vi "GetDACRS232 V1_2.vi"(3 "error in (no error)":errorcluster, 4 "VISA resource name IN":refnum<visa-resource-name>="COM1") -> (0 "error out":errorcluster, 1 "VISA resource name OUT":refnum<visa-resource-name>="COM1", 2 "DAC data out\n(hexadecimaal)":u16[](array[numeric]) format="%x")   [LabVIEW 2011]
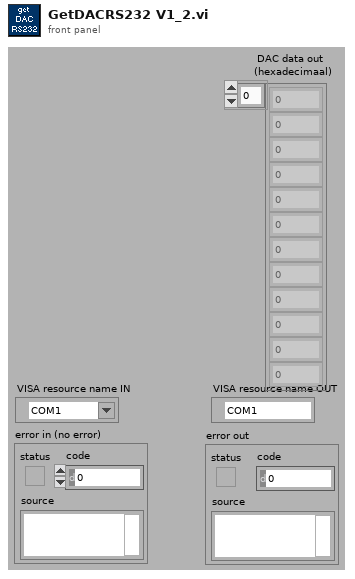
[diagram p1: front panel]
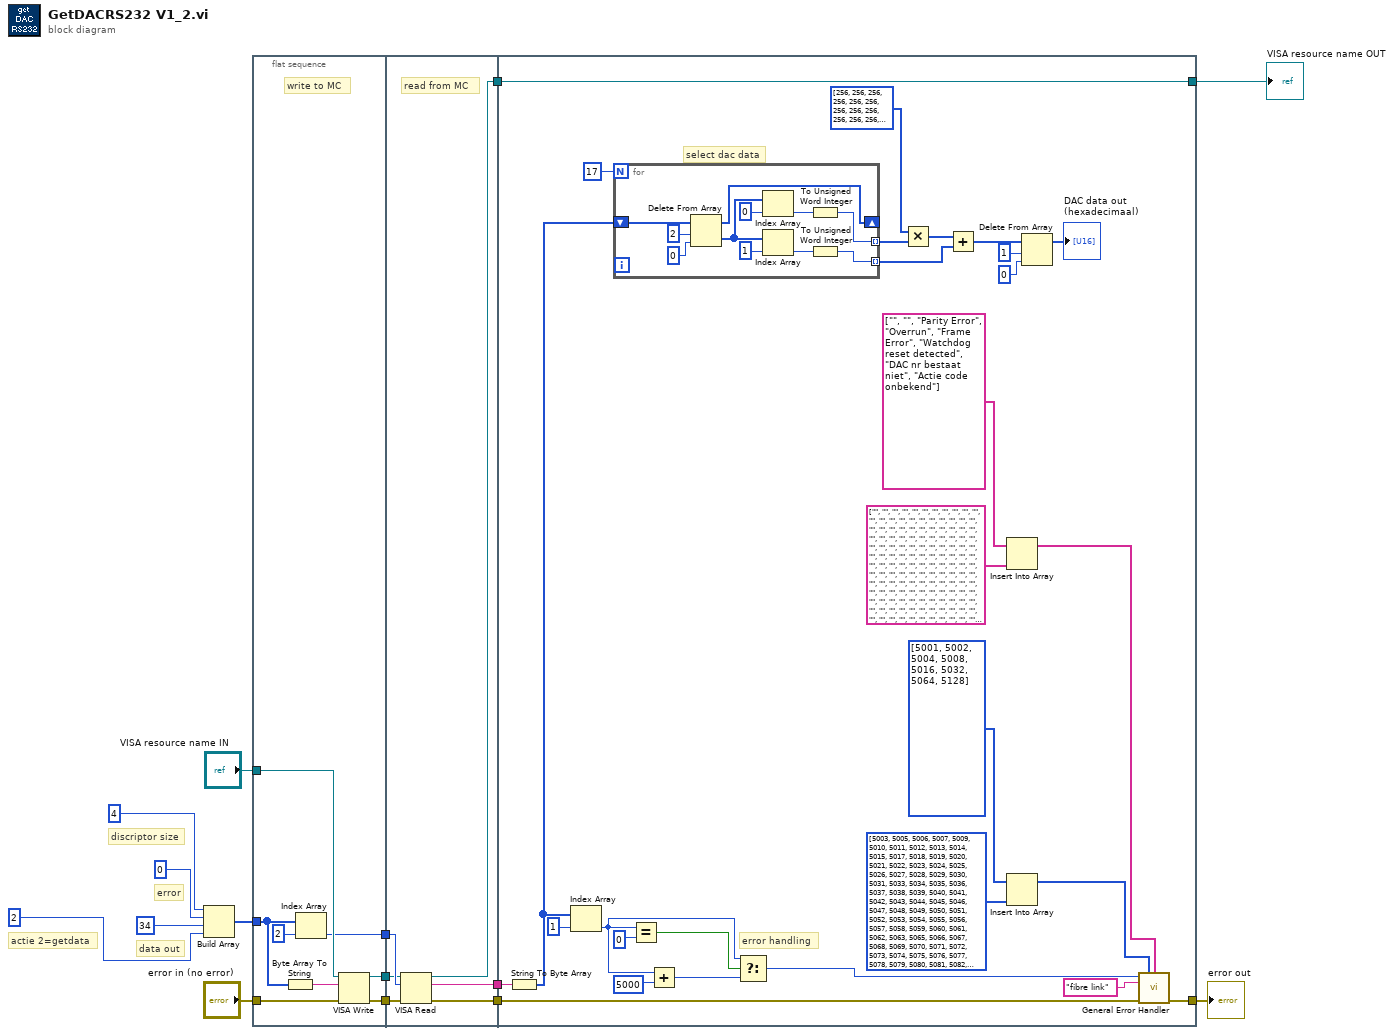
[diagram p0: block diagram]
diagram:
  # "discriptor size"
  # "error"
  # "data out"
  # "actie 2=getdata"
  n1 = Build Array(u8 4 ("array"), u8 0 ("element"), u8 34 ("element"), u8 2 ("element")) -> (w8:u8[])
  n2 = flat-sequence {
    tunnel: "VISA resource name IN" -> [w22]
    tunnel: [w20] -> w15
    tunnel: [w17] -> w14
    tunnel: [w18] -> w13
    tunnel: w8 -> [w19]
    tunnel: "error in (no error)" -> [w16]
    tunnel: w15 -> [w29]
    tunnel: w14 -> [w28]
    tunnel: w13 -> [w27]
    tunnel: [w26] -> w5
    tunnel: [w25] -> w4
    tunnel: [w24] -> w3
    tunnel: [w38] -> w1
    tunnel: w5 -> [w41]
    tunnel: w4 -> [w40]
    tunnel: [w39] -> w2
    tunnel: w3 -> [w39]
    frame #0 {
      # "write to MC"
      n3 = Byte Array To String(unsigned byte array=w19) -> (string=w23:string)
      n4 = Index Array(array=w19, index=2) -> (element=w20:u8)
      n5 = VISA Write(VISA resource name=w22, write buffer=w23, error in (no error)=w16) -> (VISA resource name out=w17:refnum<visa-resource-name>, error out=w18:errorcluster)  [unwired: 1 out]
    }
    frame #1 {
      # "read from MC"
      n6 = VISA Read(VISA resource name=w28, byte count=w29, error in (no error)=w27) -> (VISA resource name out=w24:refnum<visa-resource-name>, read buffer=w25:string, error out=w26:errorcluster)  [unwired: 1 out]
    }
    frame #2 {
      # "select dac data"
      # "error handling"
      n7 = String To Byte Array(string=w40) -> (unsigned byte array=w37:u8[])
      n8 = Index Array(array=w37, index=1) -> (element=w56:u8)
      n9 = for {
        N: 17 -> [_]
        shift-right: [w62] -> _
        shift-left: w37 -> [w66]
        tunnel: [w61] -> w45 mode=indexing
        tunnel: [w58] -> w42 mode=indexing
        n10 = Delete From Array(array=w66, length=2, index=0) -> (deleted portion=w64:u8[], array with subset deleted=w62:u8[])
        n11 = Index Array(array=w64, index=0) -> (element=w59:u8)
        n12 = Index Array(array=w64, index=1) -> (element=w60:u8)
        n13 = To Unsigned Word Integer(number=w59) -> (unsigned 16bit integer=w58:u16)
        n14 = To Unsigned Word Integer(number=w60) -> (unsigned 16bit integer=w61:u16)
      }
      n15 = Equal?(x=w56, y=u8 0) -> (x = y?=w55:bool)
      n16 = Add(x=w56, y=u32 5000) -> (x+y=w53:u32)
      n17 = Select(t=w56, s=w55, f=w53) -> (s? t:f=w54:u32)
      n18 = Multiply(x=u16[] [256, 256, 256, 256, 256, 256, 256, 256, 256, 256, 256, 256, 256, 256, 256, 256, 256], y=w42) -> (x*y=w44:u16[])
      n19 = Add(x=w44, y=w45) -> (x+y=w46:u16[])
      n20 = Insert Into Array(array=string[] ["", "", "Parity Error", "Overrun", "Frame Error", "Watchdog reset detected", "DAC nr bestaat niet", "Actie code onbekend"] ("[user-defined descriptions]"), new element=string[] ["", "", "", "", "", "", "", "", "", "", "", "", "", "", "", "", "", "", "", "", "", "", "", "", "", "", "", "", "", "", "", "", "", "", "", "", "", "", "", "", "", "", "", "", "", "", "", "", "", "", "", "", "", "", "", "", "", "", "", "", "", "", "", "", "", "", "", "", "", "", "", "", "", "", "", "", "", "", "", "", "", "", "", "", "", "", "", "", "", "", "", "", "", "", "", "", "", "", "", "", "", "", "", "", "", "", "", "", "", "", "", "", "", "", "", "", "", "", "", "", "", "", "", "", "", "", "", "", "", "", "", "", "", "", "", "", "", "", "", "", "", "", "", "", "", "", "", "", "", "", "", "", "", "", "", "", "", "", "", "", "", "", "", "", "", "", "", "", "", "", "", "", "", "", "", "", "", "", "", "", "", "", "", "", "", "", "", "", "", "", "", "", "", "", "", "", "", "", "", "", "", "", "", "", "", "", "", "", "", "", "", "", "", "", "", "", "", "", "", "", "", "", "", "", "", "", "", "", "", "", "", "", "", "", "", "", "", "", "", "", "", "", "", "", "", "", "", "", "", "", "", "", "", "", "", "", "", "", "", "", "", "", "", "", "", "", "", "", "", "", "", "", "", "", "", "", "", "", "", "", "", "", "", "", "", "", "", "", "", "", "", "", "", "", "", "", "", "", ""] ("Array 2")) -> (w30:string[])  [unwired: 1 in]
      n21 = Insert Into Array(array=i32[] [5001, 5002, 5004, 5008, 5016, 5032, 5064, 5128] ("[user-defined codes]"), new element=i32[] [5003, 5005, 5006, 5007, 5009, 5010, 5011, 5012, 5013, 5014, 5015, 5017, 5018, 5019, 5020, 5021, 5022, 5023, 5024, 5025, 5026, 5027, 5028, 5029, 5030, 5031, 5033, 5034, 5035, 5036, 5037, 5038, 5039, 5040, 5041, 5042, 5043, 5044, 5045, 5046, 5047, 5048, 5049, 5050, 5051, 5052, 5053, 5054, 5055, 5056, 5057, 5058, 5059, 5060, 5061, 5062, 5063, 5065, 5066, 5067, 5068, 5069, 5070, 5071, 5072, 5073, 5074, 5075, 5076, 5077, 5078, 5079, 5080, 5081, 5082, 5083, 5084, 5085, 5086, 5087, 5088, 5089, 5090, 5091, 5092, 5093, 5094, 5095, 5096, 5097, 5098, 5099, 5100, 5101, 5102, 5103, 5104, 5105, 5106, 5107, 5108, 5109, 5110, 5111, 5112, 5113, 5114, 5115, 5116, 5117, 5118, 5119, 5120, 5121, 5122, 5123, 5124, 5125, 5126, 5127, 5129, 5130, 5131, 5132, 5133, 5134, 5135, 5136, 5137, 5138, 5139, 5140, 5141, 5142, 5143, 5144, 5145, 5146, 5147, 5148, 5149, 5150, 5151, 5152, 5153, 5154, 5155, 5156, 5157, 5158, 5159, 5160, 5161, 5162, 5163, 5164, 5165, 5166, 5167, 5168, 5169, 5170, 5171, 5172, 5173, 5174, 5175, 5176, 5177, 5178, 5179, 5180, 5181, 5182, 5183, 5184, 5185, 5186, 5187, 5188, 5189, 5190, 5191, 5192, 5193, 5194, 5195, 5196, 5197, 5198, 5199, 5200, 5201, 5202, 5203, 5204, 5205, 5206, 5207, 5208, 5209, 5210, 5211, 5212, 5213, 5214, 5215, 5216, 5217, 5218, 5219, 5220, 5221, 5222, 5223, 5224, 5225, 5226, 5227, 5228, 5229, 5230, 5231, 5232, 5233, 5234, 5235, 5236, 5237, 5238, 5239, 5240, 5241, 5242, 5243, 5244, 5245, 5246, 5247, 5248, 5249, 5250, 5251, 5252, 5253, 5254, 5255, 5256, 5257, 5258, 5259, 5260, 5261, 5262, 5263, 5264, 5265, 5266, 5267, 5268, 5269, 5270, 5271, 5272, 5273, 5274, 5275, 5276, 5277, 5278, 5279, 5280, 5281, 5282, 5283, 5284, 5285, 5286, 5287, 5288, 5289, 5290, 5291, 5292, 5293, 5294, 5295, 5296, 5297, 5298, 5299] ("Array")) -> (w34:i32[])  [unwired: 1 in]
      n22 = Delete From Array(array=w46, length=1, index=0) -> (array with subset deleted=→"DAC data out\n(hexadecimaal)":u16[])  [unwired: 1 out]
      n23 = call <vilib>:"General Error Handler.vi"("[error code] (0)"=w54, "[user-defined codes]"=w34, "[user-defined descriptions]"=w30, "[error source] (\" \")"="fibre link" ("[error source] (\" \")"), "error in (no error)"=w41) -> ("error out"=w38:errorcluster)  [unwired: 6 in, 4 out]
    }
  }
  "error out" <- w1
  "VISA resource name OUT" <- w2
